vi "send_ThrottleSteering.vi"(4 "Counter":i32, 5 "200/freq":i32=4, 6 "Active":bool, 7 "CAN ID":u32=560 format="%x", 8 "Message":T2 {"APPS2" scale=0.0..100.0; "APPS1" scale=0.0..100.0; "Steering Angle 2" scale=90.0..-90.0; "Steering Angle 1" scale=90.0..-90.0}, 11 "CAN frame":T1[](array[typedef]) {"Data" format="%.0x"; "ArbitrationId" format="%.0x"; "Timestamp" format="%<%I:%M:%S%3u %p\n%m/%d/%Y>T"}) -> (3 "CAN frame out":T1[](array[typedef]) {"Data" format="%.0x"; "ArbitrationId" format="%.0x"; "Timestamp" format="%<%I:%M:%S%3u %p\n%m/%d/%Y>T"})   [LabVIEW 2017]
uses:
  <vilib>/nican/nican.llb/CanFrameTimed.ctl
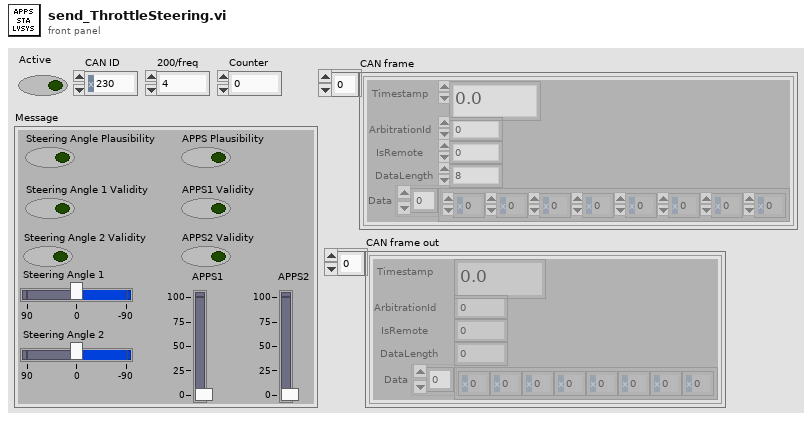
[diagram p1: front panel]
types:
  T1 = typedef "CanFrameTimed.ctl" = cluster{"Timestamp":dbl, "ArbitrationId":u32, "IsRemote":u8, "DataLength":u8, "Data":u8[]}
  T2 = cluster{"APPS Plausibility":bool, "Steering Angle 1":dbl, "Steering Angle 2":dbl, "APPS1":dbl, "APPS2":dbl, "APPS1 Validity":bool, "APPS2 Validity":bool, "Steering Angle Plausibility":bool, "Steering Angle 1 Validity":bool, "Steering Angle 2 Validity":bool}
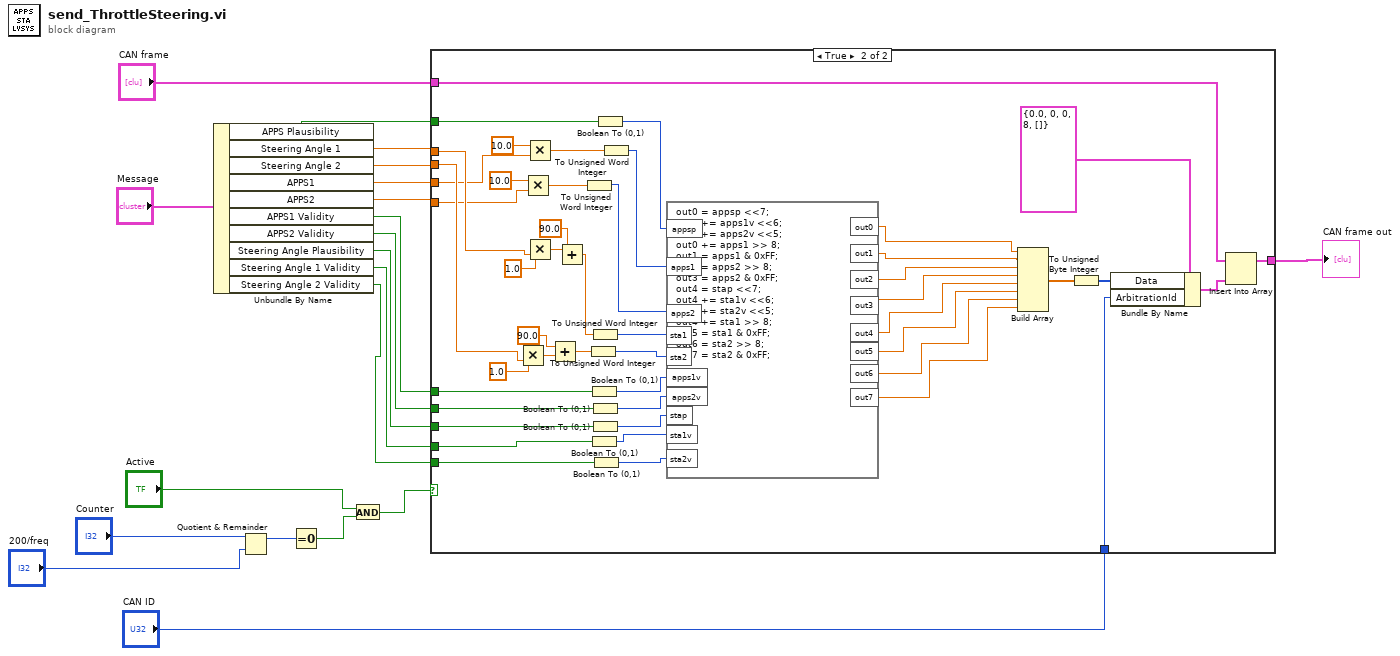
[diagram p0: block diagram]
diagram:
  n1 = Unbundle By Name("Message") -> ("APPS Plausibility"=w15:bool, "Steering Angle 1"=w18:dbl, "Steering Angle 2"=w19:dbl, "APPS1"=w17:dbl, "APPS2"=w16:dbl, "APPS1 Validity"=w14:bool, "APPS2 Validity"=w12:bool, "Steering Angle Plausibility"=w13:bool, "Steering Angle 1 Validity"=w11:bool, "Steering Angle 2 Validity"=w10:bool)
  n2 = Quotient & Remainder(x="Counter", y="200/freq") -> (x-y*floor(x/y)=w5:i32)  [unwired: 1 out]
  n3 = Equal To 0?(x=w5) -> (x = 0?=w3:bool)
  n4 = And(x="Active", y=w3) -> (x .and. y?=w2:bool)
  n5 = case shown="True" w2 {
    tunnel: w19 -> [_ w52]
    tunnel: w18 -> [_ w51]
    tunnel: w17 -> [_ w50]
    tunnel: w16 -> [_ w49]
    tunnel: w15 -> [_ w48]
    tunnel: w14 -> [_ w46]
    tunnel: w13 -> [_ w45]
    tunnel: w12 -> [_ w44]
    tunnel: w11 -> [_ w43]
    tunnel: w10 -> [_ w42]
    tunnel: "CAN frame" -> [w21 w25]
    tunnel: [w21 w23] -> w8
    tunnel: "CAN ID" -> [_ w22]
    frame False {
    }
    frame True {
      n6 = Multiply(x=1.0, y=w52) -> (x*y=w62:dbl)
      n7 = Multiply(x=10.0, y=w49) -> (x*y=w59:dbl)
      n8 = Multiply(x=10.0, y=w50) -> (x*y=w60:dbl)
      n9 = Multiply(x=1.0, y=w51) -> (x*y=w64:dbl)
      n10 = Add(x=90.0, y=w62) -> (x+y=w57:dbl)
      n11 = Add(x=w64, y=90.0) -> (x+y=w58:dbl)
      n12 = To Unsigned Word Integer(number=w59) -> (unsigned 16bit integer=w54:u16)
      n13 = To Unsigned Word Integer(number=w57) -> (unsigned 16bit integer=w56:u16)
      n14 = Boolean To (0,1)(Boolean=w46) -> (0, 1=w41:i16)
      n15 = Boolean To (0,1)(Boolean=w43) -> (0, 1=w38:i16)
      n16 = To Unsigned Word Integer(number=w58) -> (unsigned 16bit integer=w55:u16)
      n17 = Boolean To (0,1)(Boolean=w44) -> (0, 1=w40:i16)
      n18 = Boolean To (0,1)(Boolean=w45) -> (0, 1=w39:i16)
      n19 = Boolean To (0,1)(Boolean=w42) -> (0, 1=w37:i16)
      n20 = Boolean To (0,1)(Boolean=w48) -> (0, 1=w47:i16)
      n21 = To Unsigned Word Integer(number=w60) -> (unsigned 16bit integer=w53:u16)
      n22 = formula code="out0 = appsp <<7;\nout0 += apps1v <<6;\nout0 += apps2v <<5;\nout0 += apps1 >> 8;\nout1 = apps1 & 0xFF;\nout2 = apps2 >> 8;\nout3 = apps2 & 0xFF;\nout4 = stap <<7;\nout4 += sta1v <<6;\nout4 += sta2v <<5;\nout4 += sta1 >> 8;\nout5 = sta1 & 0xFF;\nout6 = sta2 >> 8;\nout7 = sta2 & 0xFF;"("apps1"=w53, "apps2"=w54, "sta1"=w55, "sta2"=w56, "appsp"=w47, "apps1v"=w41, "apps2v"=w40, "stap"=w39, "sta1v"=w38, "sta2v"=w37) -> ("out1"=w35:dbl, "out2"=w34:dbl, "out3"=w33:dbl, "out0"=w36:dbl, "out4"=w32:dbl, "out5"=w31:dbl, "out6"=w30:dbl, "out7"=w29:dbl)
      n23 = Build Array(w36, w35, w34, w33, w32, w31, w30, w29) -> (w28:dbl[])
      n24 = To Unsigned Byte Integer(number=w28) -> (unsigned 8bit integer=w27:u8[])
      n25 = Bundle By Name(cluster=T1 {"Timestamp"=0.0, "ArbitrationId"=0, "IsRemote"=0, "DataLength"=8, "Data"=[]} ("CAN frame"), "Data"=w27, "ArbitrationId"=w22) -> (w24:T1)
      n26 = Insert Into Array(array=w25, new element=w24) -> (w23:T1[])  [unwired: 1 in]
    }
  }
  "CAN frame out" <- w8
